vi "Push.vi"(10 "Element":T1, 11 "TypedCircularBuffer in":refnum<class "TypedCircularBuffer.lvclass">) -> (1 "overflow?":bool, 2 "overflow element":T1, 3 "TypedCircularBuffer out":refnum<class "TypedCircularBuffer.lvclass">)   [LabVIEW 2024, in "TypedCircularBuffer.lvclass"]
uses:
  TypedCircularBuffer.lvclass
  Type.ctl
  TypedCircularBuffer.lvclass/TypedCircularBuffer.ctl
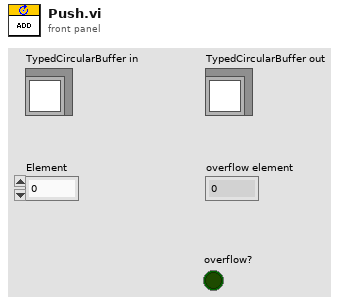
[diagram p1: front panel]
types:
  T1 = typedef "TypedCircularBuffer.lvclass/Type.ctl" = i32
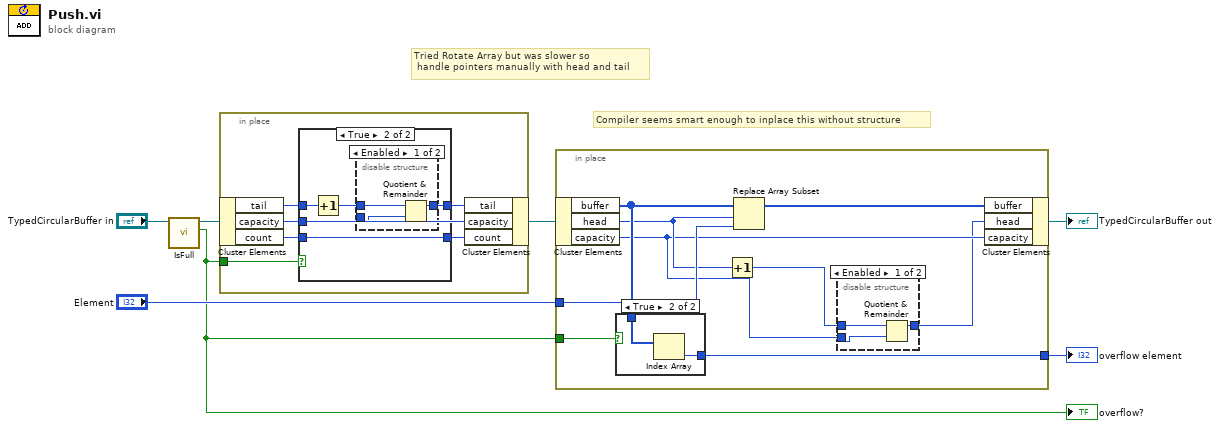
[diagram p0: block diagram]
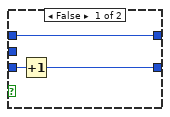
[diagram p2: hidden frame]
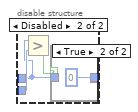
[diagram p3: hidden frame]
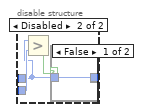
[diagram p5: hidden frame]
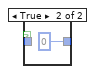
[diagram p6: hidden frame]
diagram:
  # "Compiler seems smart enough to inplace this without structure"
  # "Tried Rotate Array but was slower so\n handle pointers manually with head and tail"
  n1 = call "IsFull.vi"("TypedCircularBuffer in"="TypedCircularBuffer in") -> ("Full?"=w1:bool, "TypedCircularBuffer out"=w3:refnum<class "TypedCircularBuffer.lvclass">)  [unwired: 9 in]
  "overflow?" <- w1
  n2 = in-place {
    in-place-border: w1 -> [w8]
    n3 = in-place-cluster #1(w3) -> ("tail"=w13:u32, "capacity"=w10:u32, "count"=w9:u32)
    n4 = case shown="True" w8 {
      tunnel: w13 -> [w16 w20]
      tunnel: w10 -> [_ w19]
      tunnel: [w16 w18] -> w12
      tunnel: w9 -> [w15 w17]
      tunnel: [w14 w17] -> w11
      frame False {
        n5 = Increment(x=w15) -> (x+1=w14:u32)
      }
      frame True {
        n6 = Increment(x=w20) -> (x+1=w21:u32)
        n7 = disable-structure shown="Enabled" {
          disable-tunnel: w21 -> [w24 w25]
          disable-tunnel: w19 -> [w23 w28]
          disable-tunnel: [w22 w26] -> w18
          frame Enabled {
            n8 = Quotient & Remainder(x=w24, y=w23) -> (x-y*floor(x/y)=w22:u32)  [unwired: 1 out]
          }
          frame Disabled {
            n9 = Greater?(x=w25, y=w28) -> (0:w27:bool)
            n10 = case shown="True" w27 {
              tunnel: [w29 u32 0] -> w26
              tunnel: w25 -> [w29 _]
              frame False {
              }
              frame True {
              }
            }
          }
        }
      }
    }
    n11 = in-place-cluster #1("tail"=w12, "capacity"=w10, "count"=w11) -> (w4:refnum<class "TypedCircularBuffer.lvclass">)
  }
  n12 = in-place {
    in-place-border: "Element" -> [w36]
    in-place-border: [w34] -> w2
    in-place-border: w1 -> [w38]
    n13 = in-place-cluster #2(w4) -> ("buffer"=w37:T1[], "head"=w35:u32, "capacity"=w33:u32)
    n14 = case shown="True" w38 {
      tunnel: w37 -> [_ w50]
      tunnel: [_ w49] -> w34
      frame False {
      }
      frame True {
        n15 = Index Array(array=w50) -> (element=w49:T1)  [unwired: 1 in]
      }
    }
    n16 = Increment(x=w35) -> (x+1=w32:u32)
    n17 = Replace Array Subset(array=w37, new element=w36, index=w35) -> (w39:T1[])
    n18 = disable-structure shown="Enabled" {
      disable-tunnel: w32 -> [w42 w43]
      disable-tunnel: w33 -> [w41 w46]
      disable-tunnel: [w40 w44] -> w31
      frame Enabled {
        n19 = Quotient & Remainder(x=w42, y=w41) -> (x-y*floor(x/y)=w40:u32)  [unwired: 1 out]
      }
      frame Disabled {
        n20 = Greater?(x=w43, y=w46) -> (0:w45:bool)
        n21 = case shown="False" w45 {
          tunnel: [w47 u32 0] -> w44
          tunnel: w43 -> [w47 _]
          frame False {
          }
          frame True {
          }
        }
      }
    }
    n22 = in-place-cluster #2("buffer"=w39, "head"=w31, "capacity"=w33) -> (→"TypedCircularBuffer out":refnum<class "TypedCircularBuffer.lvclass">)
  }
  "overflow element" <- w2
